vi "CRYInit RunIndex.vi"(10 "Steps In":T1[](array[typedef]) {"Repeat State Array"."Start" format="%#_5g"; "Y dB ref" format="%.1f"; "Y data" items=["dB", "Lin"]; "Start" format="%#_5g"}) -> ()   [LabVIEW 2013]
uses:
  Typedef Control/CRYStep.ctl
  CRYStatistics Global.vi
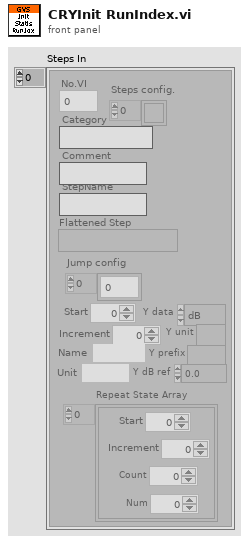
[diagram p1: front panel]
types:
  T1 = typedef "CRYStep.ctl" = cluster{"No.VI":i32, "Category":string, "StepName":string, "Seq setup flattened":string, "Comment":string, "Steps config.":bool[], "Jump config":i32[], "Start":dbl, "Increment":dbl, "Name":string, "Unit":string, "Y data":u16, "Y prefix":string, "Y dB ref":dbl, "Y unit":string, "Repeat State Array":cluster{"Start":dbl, "Increment":dbl, "Count":i32, "Num":i32}[]}
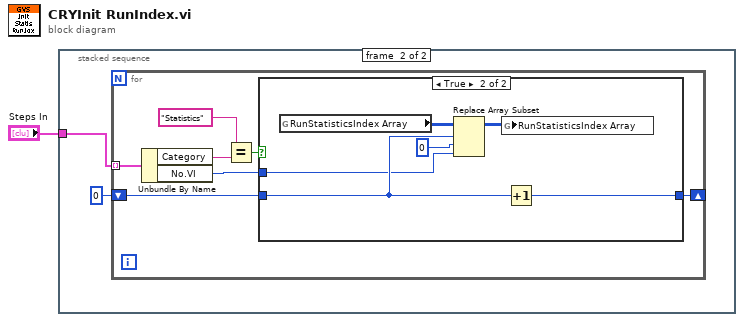
[diagram p0: block diagram]
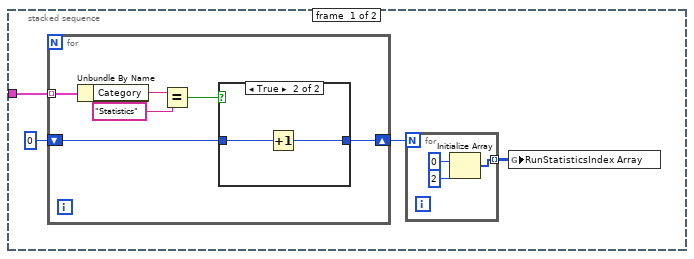
[diagram p2: hidden frame]
diagram:
  n1 = stacked-sequence {
    tunnel: "Steps In" -> [w2 w19]
    frame #0 {
      n2 = for {
        tunnel: w2 -> [w11] mode=indexing
        shift-right: [w6] -> w3
        shift-left: i16 0 -> [w7]
        n3 = Unbundle By Name(w11) -> ("Category"=w10:string)
        n4 = Equal?(x=w10, y="Statistics") -> (x = y?=w8:bool)
        n5 = case shown="True" w8 {
          tunnel: w7 -> [w12 w14]
          tunnel: [w12 w13] -> w6
          frame False {
          }
          frame True {
            n6 = Increment(x=w14) -> (x+1=w13:i16)
          }
        }
      }
      n7 = for {
        N: w3 -> [_]
        tunnel: [w15] -> w5 mode=indexing
        n8 = Initialize Array(i16 0 ("element"), 2 ("dimension size")) -> (w15:i16[])
      }
      n9 = global write "CRYStatistics Global.vi" "RunStatisticsIndex Array"(w5) -> ()
    }
    frame #1 {
      n10 = for {
        tunnel: w19 -> [w26] mode=indexing
        shift-right: [w23] -> _
        shift-left: i16 0 -> [w24]
        n11 = Unbundle By Name(w26) -> ("Category"=w22:string, "No.VI"=w20:i32)
        n12 = Equal?(x="Statistics" ("y"), y=w22) -> (x = y?=w25:bool)
        n13 = case shown="True" w25 {
          tunnel: w24 -> [w27 w30]
          tunnel: [w27 w33] -> w23
          tunnel: w20 -> [_ w29]
          frame False {
          }
          frame True {
            n14 = global read "CRYStatistics Global.vi" "RunStatisticsIndex Array"() -> (w32:u16[][])
            n15 = Replace Array Subset(array=w32, new element=w29, index (row)=w30, index (col)=0 ("disabled index (col)")) -> (w28:u16[][])
            n16 = global write "CRYStatistics Global.vi" "RunStatisticsIndex Array"(w28) -> ()
            n17 = Increment(x=w30) -> (x+1=w33:i16)
          }
        }
      }
    }
  }
